vi "what is alive.vi"() -> (0 "nodes alive":string[](array[string]))   [LabVIEW 2020, in "Publisher Subscriber.lvlib"]
uses:
  Publisher Subscriber.lvlib
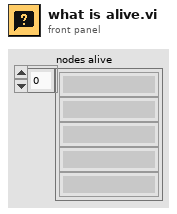
[diagram p1: front panel]
types:
  T1 = cluster{"subscription map ref":refnum<data-value>, "variable dvr refs":refnum<data-value>}
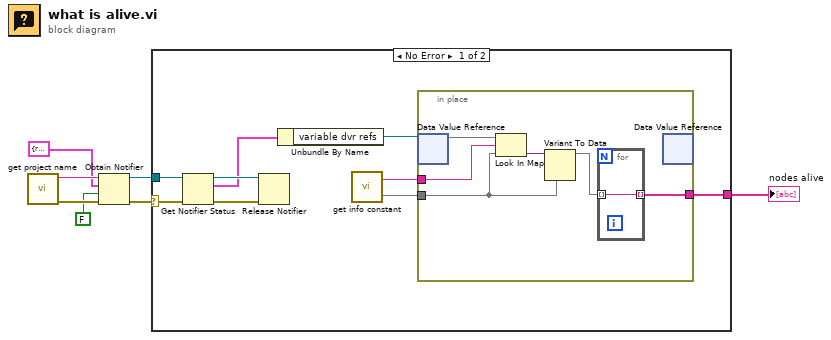
[diagram p0: block diagram]
diagram:
  n1 = call "get project name.vi"() -> ("error out"=w4:errorcluster, "Project name"=w5:string)  [unwired: 10 in]
  n2 = Obtain Notifier(name (unnamed)=w5, notification data type=T1 {"subscription map ref"=refnum, "variable dvr refs"=refnum} ("Cluster"), create if not found? (T)=FALSE, error in (no error)=w4) -> (notifier out=w6:refnum<notifier>, error out=w7:errorcluster)  [unwired: 1 out]
  n3 = case shown="No Error" w7 {
    selector: w7 -> [w16 _]
    tunnel: w6 -> [w15 _]
    tunnel: [w10 _] -> w3
    frame No Error {
      n4 = Get Notifier Status(notifier=w15, error in (no error)=w16) -> (notifier out=w14:refnum<notifier>, current notification=w12:T1, error out=w13:errorcluster)  [unwired: 2 out]
      n5 = Release Notifier(notifier=w14, error in (no error)=w13) -> ()  [unwired: 1 in, 3 out]
      n6 = Unbundle By Name(w12) -> ("variable dvr refs"=w11:refnum<data-value>)
      n7 = call "get info constant.vi"() -> ("set"=w8:set{string}, "String"=w9:string)  [unwired: 4 in]
      n8 = in-place {
        in-place-border: w9 -> [w21]
        in-place-border: [w19] -> w10
        in-place-border: w8 -> [w17]
        n9 = in-place-dvr #1(w11) -> (w22:map{string, variant})  [unwired: 1 out]
        n10 = Look In Map(map=w22, key=w21, default value=w17) -> (value=w20:variant)  [unwired: 1 out]
        n11 = Variant To Data(type=w17, Variant=w20) -> (data=w18:set{string})  [unwired: 1 in, 1 out]
        n12 = for {
          tunnel: [w23] -> w19 mode=indexing
          tunnel: w18 -> [w23] mode=indexing
        }
        n13 = in-place-dvr #1() -> ()  [unwired: 1 in, 2 out]
      }
    }
    frame Error {
    }
  }
  "nodes alive" <- w3
